vi "Set Target Velocity.vi"(0 "reference in":refnum<class "SmartMotor.lvclass">, 2 "Target Velocity (RPM)":dbl, 5 "error in (no error)":errorcluster) -> (14 "reference out":refnum<class "SmartMotor.lvclass">, 19 "error out":errorcluster)   [LabVIEW 2017, in "SmartMotor.lvclass"]
uses:
  SmartMotor.lvclass
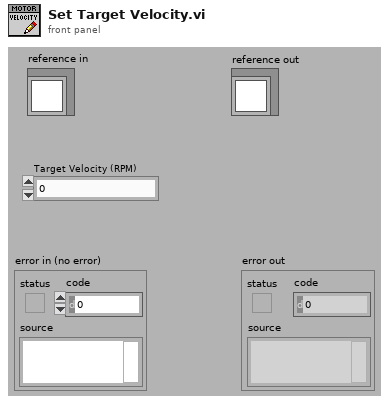
[diagram p1: front panel]
types:
  T1 = typedef "SmartMotor.lvclass/ObjectAttributes.ctl" = cluster{"SmartMotor Chain VISA Resource":refnum<visa-resource-name>, "SmartMotor Chain Address":i16, "Motor Absolute Position":i32, "Motor Relative Position":i32, "Motor Torque":i32, "Motor Voltage":i32, "Screwdriver Engaged":bool, "Screwdriver Torque Limit":i32, "Torque Monitor On/Off Status":bool, "Torque Monitor VI Reference":refnum<vi>, "Absolute Motor Torque (Filtered)":dbl, "SmartMotor Status":T2, "SmartMotor Error":T3}
  T2 = typedef "SmartMotor.lvclass/SmartMotor Status.ctl" = enum8{"Stopped", "Moving"}
  T3 = typedef "SmartMotor.lvclass/SmartMotor Error.ctl" = enum8{"None", "Read Error", "Low Voltage"}
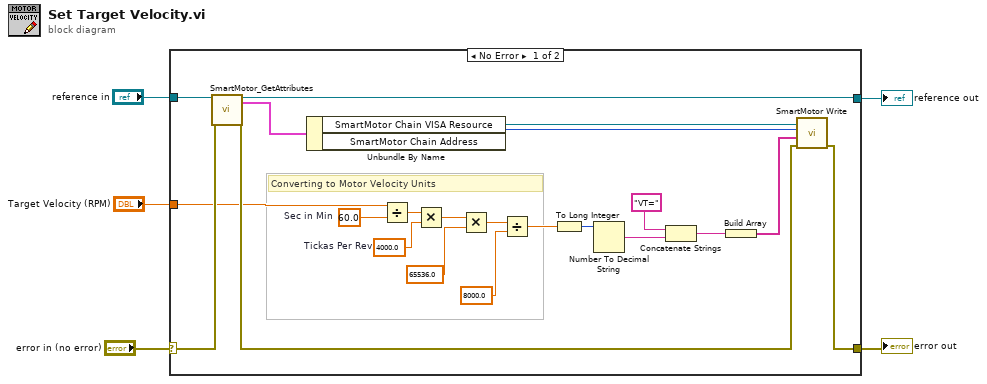
[diagram p0: block diagram]
diagram:
  n1 = case shown="No Error" "error in (no error)" {
    selector: "error in (no error)" -> [w26 w29]
    tunnel: [w6 w29] -> w4
    tunnel: [w25 w28] -> w2
    tunnel: "reference in" -> [w27 w28]
    tunnel: "Target Velocity (RPM)" -> [w23 _]
    frame No Error {
      w18 = 4000.0  # Tickas Per Rev
      w20 = 60.0  # Sec in Min
      # "Converting to Motor Velocity Units"
      n2 = call "SmartMotor_GetAttributes.vi"("reference in"=w27, "error in (no error)"=w26) -> ("reference out"=w25:refnum<class "SmartMotor.lvclass">, "Data"=w7:T1, "error out"=w24:errorcluster)  [unwired: 14 in, 1 out]
      n3 = Unbundle By Name(w7) -> ("SmartMotor Chain VISA Resource"=w22:refnum<visa-resource-name>, "SmartMotor Chain Address"=w8:i16)
      n4 = Divide(x=w23, y=w20) -> (x/y=w19:dbl)
      n5 = Multiply(x=w19, y=w18) -> (x*y=w17:dbl)
      n6 = Multiply(x=w17, y=65536.0) -> (x*y=w15:dbl)
      n7 = Divide(x=w15, y=8000.0) -> (x/y=w13:dbl)
      n8 = To Long Integer(number=w13) -> (32bit integer=w12:i32)
      n9 = Number To Decimal String(number=w12) -> (decimal integer string=w10:string)  [unwired: 1 in]
      n10 = Concatenate Strings("VT=", w10) -> (w21:string)
      n11 = Build Array(w21) -> (w9:string[])
      n12 = call "SmartMotor Write.vi"("VISA resource IN"=w22, "Motor Number"=w8, "Motor Command Array"=w9, "Error In"=w24) -> ("Error Out"=w6:errorcluster)  [unwired: 3 in, 2 out]
    }
    frame Error {
    }
  }
  "error out" <- w4
  "reference out" <- w2
